vi "面积.vi"(8 "error in (no error)":errorcluster caption="错误输入（无错误）", 11 "圆形 输入":refnum<class "圆形.lvclass"> caption="DNL_LabVIEW Object in") -> (0 "error out":errorcluster caption="错误输出", 2 "面积":dbl, 3 "圆形 输出":refnum<class "圆形.lvclass"> caption="DNL_LabVIEW Object out")   [LabVIEW 2013, in "圆形.lvclass"]
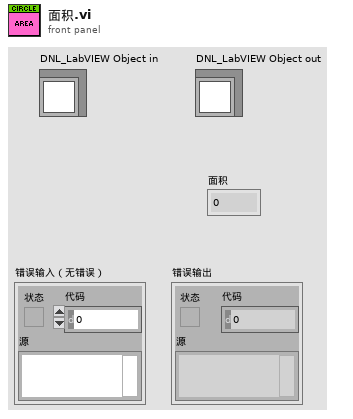
[diagram p1: front panel]
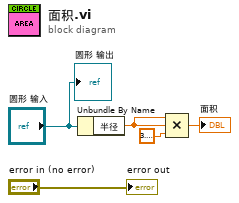
[diagram p0: block diagram]
diagram:
  n1 = Unbundle By Name("圆形 输入") -> ("半径"=w4:dbl)
  n2 = Compound Arithmetic op=MULTIPLY(w4, w4, 3.141592653589793) -> (→"面积":dbl)
  "error out" <- "error in (no error)"
  "圆形 输出" <- "圆形 输入"
